vi "Balance Loop.vi"(8 "error in (no error)":errorcluster, 9 "PID gains":T1={"proportional gain (Kc)"=-4.805, "integral time (Ti, min)"=50.38629, "derivative time (Td, min)"=0.000943} {"derivative time (Td, min)" format="%.3f"; "integral time (Ti, min)" format="%.3f"; "proportional gain (Kc)" format="%.3f"}, 10 "maxDiff":dbl=0.75, 11 "Refnum in":refnum<k20>) -> (0 "error out":errorcluster, 3 "Refnum Out":refnum<k20>)   [LabVIEW 2016]
uses:
  <vilib>/Platform/TimedLoop/XDataNode/timing_clust.ctl
  <vilib>/Platform/TimedLoop/XDataNode/nitl_modes.ctl
  <vilib>/Platform/TimedLoop/XDataNode/wakeup.ctl
  Typedef/Remote Control Cluster.ctl
  Typedef/INS Data.ctl
  Shared resoruces/Navigation Variables.vi
  Shared resoruces/Front Panel Control Variables.vi
  <vilib>/addons/control/pid/pid.llb/PID (DBL).vi
  <vilib>/Utility/error.llb/Error Cluster From Error Code.vi
  <vilib>/rvi/errors/niLvFpgaAdjustHostInterfaceError.vi
  <vilib>/RVI Host/nirviSupport.llb/nirviErrorClusterFromErrorCode.vi
  <vilib>/platform/TimedLoop/XDataNode/XDataNode.xnode
  <vilib>/rvi/interface/nirviMethod/nirviMethod.xnode
  <vilib>/rvi/interface/nirviReadWriteControl/nirviReadWriteControl.xnode
  NiFpgaLv.dll
  <vilib>/rvi/interface/Simulation/niFpgaSimulationCallBeginRW.vi
  <vilib>/FPGAPlugInAG/Dynamic/niLvFpga_WriteFifo_Dynamic.vi
  <vilib>/rvi/errors/niLvFpgaMergeErrorWithErrorCode.vi
  <vilib>/rvi/interface/nirviMethod/StockFPGA_InlinedMethodWaitForSingleIRQ.vi
  <vilib>/FPGAPlugInAG/Dynamic/niLvFpga_WaitOnIrq_Dynamic.vi
  <vilib>/FPGAPlugInAG/Dynamic/niLvFpga_AcknowledgeIrq_Dynamic.vi
  <vilib>/addons/control/pid/NI_PID_pid.lvlib
  Shared resoruces/Shared resources RT.lvlib
  <vilib>/Platform/TimedLoop/XDataNode/XDNodeRunTimeDep.lvlib
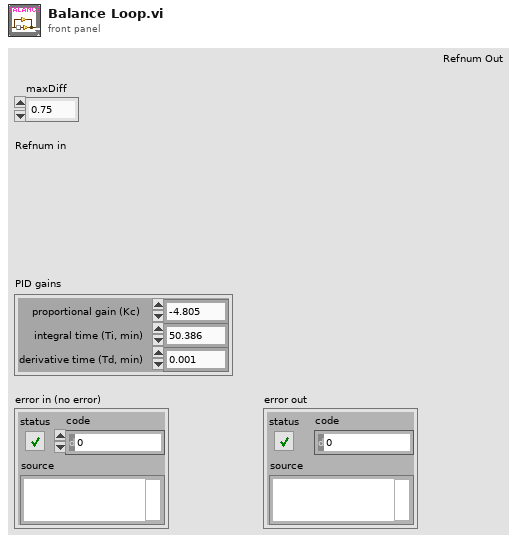
[diagram p1: front panel]
types:
  T1 = cluster{"proportional gain (Kc)":dbl, "integral time (Ti, min)":dbl, "derivative time (Td, min)":dbl}
  T2 = typedef "XDNodeRunTimeDep.lvlib/timing_clust.ctl" = cluster{"Expected End [f-1]":u64, "Actual End [f-1]":u64, "Finished Late? [f-1]":bool, "Expected End [i-1]":u64, "Actual End [i-1]":u64, "Finished Late? [i-1]":bool, "Expected Start [i]":u64, "Actual Start [i]":u64, "Expected Start [f]":u64, "Actual Start [f]":u64, "Source Name":string, "Structure Name":string, "Period":i64, "Deadline":i64, "Offset":i64, "Start":i64, "Priority":i32, "Timeout":i32, "Mode":T3, "Wakeup Reason":T4, "Error":errorcluster, "Source Type":string, "Secondary Source Type":string, "Global End Time":u64, "Global Start Time":u64, "Frame Duration":u64, "Iteration Duration":u64, "Assigned CPU":i32, "I/O Scan Engine Mode":u32}
  T3 = typedef "XDNodeRunTimeDep.lvlib/nitl_modes.ctl" = enum32{"No Change", "Process missed periods, maintain original phase", "Discard missed periods, maintain original phase", "Process missed periods, ignore original phase", "Discard missed periods, ignore original phase"}
  T4 = typedef "XDNodeRunTimeDep.lvlib/wakeup.ctl" = enum32{"Normal", "Aborted", "Asynchronous wakeup", "Timing source error", "Timed loop error", "Timeout"}
  T5 = typedef "Remote Control Cluster.ctl" = cluster{"Pot1":u16, "Pot2":u16, "Pot3":u16, "Pot4":u16, "Switch1":cluster{"L":bool, "H":bool}, "Switch2":cluster{"L":bool, "H":bool}, "Switch3":cluster{"L":bool, "H":bool}}
  T6 = typedef "INS Data.ctl" = cluster{"Yaw":sgl, "Pitch":sgl, "Roll":sgl, "Lat":dbl, "Long":dbl, "Alt":dbl, "North":dbl, "East":dbl, "Down":dbl, "PosU":dbl, "VelU":dbl}
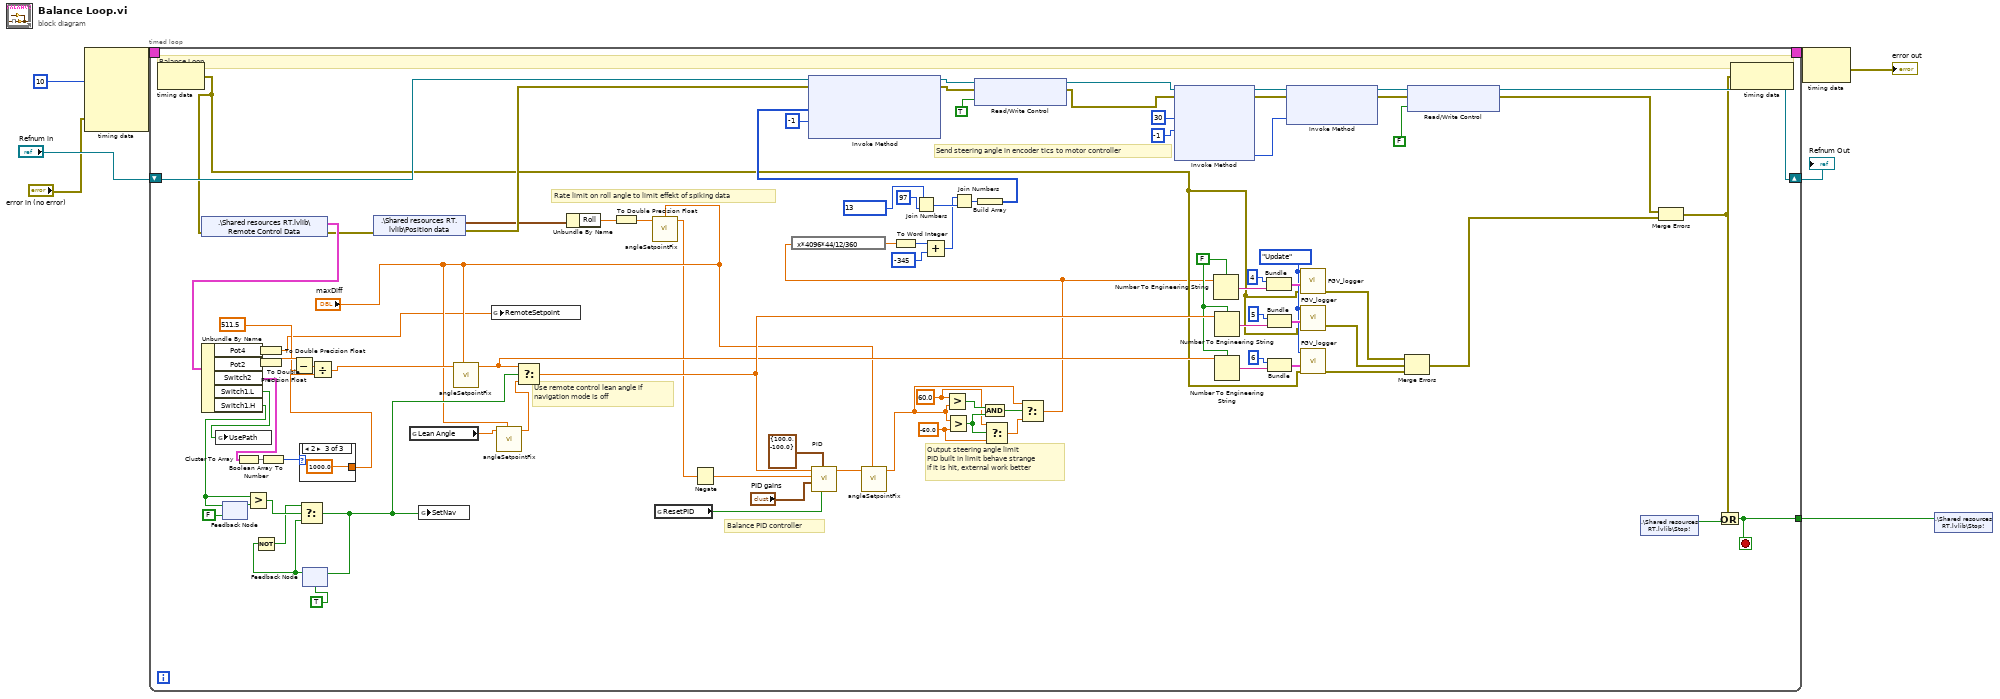
[diagram p0: block diagram]
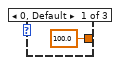
[diagram p2: hidden frame]
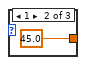
[diagram p3: hidden frame]
diagram:
  n1 = node-c288(i64 10 ("Period"), "error in (no error)") -> (w5:T2)  [unwired: 3 in]
  n2 = timed-loop {
    shift-right: [w97] -> w6
    shift-left: "Refnum in" -> [w98]
    tunnel: [w67] -> w7
    timing: w5 -> [_]
    timing-out: [_] -> w4
    stop <- w67 stop-if-true
    w17 = -60.0
    w18 = 60.0
    w28 = enum16{"Update", "Log", "Init"}."Update" ("Command")
    w32 = FALSE ("use system decimal point (T)")
    # "Use remote control lean angle if \nnavigation mode is off"
    # "Rate limit on roll angle to limit effekt of spiking data"
    # "Output steering angle limit\nPID built in limit behave strange\nif it is hit, external work better"
    # "Balance PID controller"
    # "Send steering angle in encoder tics to motor controller"
    # "Balance Loop"
    n3 = node-c288() -> (w25:errorcluster)  [unwired: 1 in]
    n4 = shared-variable ".\\Shared resources RT.lvlib\\Remote Control Data"(error in=w25) -> (w66:T5, error out=w61:errorcluster)
    n5 = Unbundle By Name(w66) -> ("Pot4"=w23:u16, "Pot2"=w96:u16, "Switch2"=w65:cluster{"L":bool, "H":bool}, "Switch1.L"=w26:bool, "Switch1.H"=w27:bool)
    n6 = global write "Navigation Variables.vi" "UsePath"(w26) -> ()
    n7 = feedback-in #1(w27) -> ()
    n8 = feedback #1(FALSE ("H")) -> (w47:bool)
    n9 = Cluster To Array(cluster=w65) -> (array=w64:bool[])
    n10 = Greater?(x=w27, y=w47) -> (0:w45:bool)
    n11 = To Double Precision Float(number=w23) -> (double precision float=w10:dbl)
    n12 = To Double Precision Float(number=w96) -> (double precision float=w94:dbl)
    n13 = Boolean Array To Number(Boolean array=w64) -> (number=w63:u32)
    n14 = Subtract(x=w94, y=511.5 ("x")) -> (x-y=w95:dbl)
    n15 = case shown="2" w63 {
      tunnel: [100.0 45.0 1000.0] -> w62
      frame 0, Default {
      }
      frame 1 {
      }
      frame 2 {
      }
    }
    n16 = feedback #2(TRUE) -> (w43:bool)
    n17 = Not(x=w43) -> (.not. x?=w42:bool)
    n18 = Select(t=w42, s=w45, f=w43) -> (s? t:f=w36:bool)
    n19 = feedback-in #2(w36) -> ()
    n20 = Divide(x=w95, y=w62) -> (x/y=w30:dbl)
    n21 = shared-variable ".\\Shared resources RT.lvlib\\Position data"(error in=w61) -> (w59:T6, error out=w60:errorcluster)
    n22 = global read "Navigation Variables.vi" "Lean Angle"() -> (w38:dbl)
    n23 = global write "Navigation Variables.vi" "SetNav"(w36) -> ()
    n24 = call "angleSetpointFix.vi"("maxDiff"="maxDiff", "Angle in"=w30) -> ("Angle out"=w29:dbl)  [unwired: 9 in]
    n25 = global write "Navigation Variables.vi" "RemoteSetpoint"(w10) -> ()
    n26 = call "angleSetpointFix.vi"("maxDiff"="maxDiff", "Angle in"=w38) -> ("Angle out"=w37:dbl)  [unwired: 9 in]
    n27 = Select(t=w29, s=w36, f=w37) -> (s? t:f=w40:dbl)
    n28 = Unbundle By Name(w59) -> ("Roll"=w14:sgl)
    n29 = To Double Precision Float(number=w14) -> (double precision float=w11:dbl)
    n30 = call "angleSetpointFix.vi"("maxDiff"="maxDiff", "Angle in"=w11) -> ("Angle out"=w12:dbl)  [unwired: 9 in]
    n31 = global read "Front Panel Control Variables.vi" "ResetPID"() -> (w39:bool)
    n32 = Negate(x=w12) -> (-x=w9:dbl)
    n33 = call-poly <vilib>:"PID.vi"("reinitialize? (F)"=w39, "output range"=cluster{"output high":dbl, "output low":dbl} {"output high"=100.0, "output low"=-100.0}, "PID gains"="PID gains", "process variable"=w9, "setpoint"=w40) -> ("output"=w69:dbl)  [unwired: 5 in, 1 out]
    n34 = call "angleSetpointFix.vi"("maxDiff"="maxDiff", "Angle in"=w69) -> ("Angle out"=w20:dbl)  [unwired: 9 in]
    n35 = Join Numbers(hi=u8 13 ("lo"), lo=u8 97) -> ((hi.lo)=w77:u16)
    n36 = Greater?(x=w18, y=w20) -> (0:w22:bool)
    n37 = Greater?(x=w20, y=w17) -> (0:w19:bool)
    n38 = And(x=w22, y=w19) -> (x .and. y?=w21:bool)
    n39 = Select(t=w18, s=w19, f=w17) -> (s? t:f=w16:dbl)
    n40 = Select(t=w20, s=w21, f=w16) -> (s? t:f=w15:dbl)
    n41 = expression code="x*4096*44/12/360"(w15) -> (w71:dbl)
    n42 = To Word Integer(number=w71) -> (16bit integer=w74:i16)
    n43 = Add(x=w74, y=i16 -345 ("hi")) -> (x+y=w72:i16)
    n44 = Join Numbers(hi=w72, lo=w77) -> ((hi.lo)=w76:u32)
    n45 = Build Array(w76) -> (w73:u32[])
    n46 = xnode "Invoke Method"("FPGA VI Reference In"=w98, "error in"=w60, "Data"=w73, "Timeout (ms)"=-1) -> ("FPGA VI Reference Out"=w85:refnum<k20>, "error out"=w86:errorcluster)  [unwired: 1 out]
    n47 = xnode "Read/Write Control"("FPGA VI Reference In"=w85, "error in"=w86, "ODrive RT Control"=TRUE) -> ("FPGA VI Reference Out"=w84:refnum<k20>, "error out"=w83:errorcluster)
    n48 = xnode "Invoke Method"("FPGA VI Reference In"=w84, "error in"=w83, "IRQ Number(s)"=30, "Timeout (ms)"=-1) -> ("FPGA VI Reference Out"=w92:refnum<k20>, "error out"=w91:errorcluster, "IRQ(s) Asserted"=w81:i32)  [unwired: 1 out]
    n49 = Number To Engineering String(1:w32, 4:w15) -> (0:w56:string)  [unwired: 2 in]
    n50 = Number To Engineering String(1:w32, 4:w40) -> (0:w53:string)  [unwired: 2 in]
    n51 = Number To Engineering String(1:w32, 4:w29) -> (0:w33:string)  [unwired: 2 in]
    n52 = Bundle(4, w56) -> (w57:cluster{i32, string})  [unwired: 1 in]
    n53 = Bundle(5, w53) -> (w54:cluster{i32, string})  [unwired: 1 in]
    n54 = Bundle(6, w33) -> (w34:cluster{i32, string})  [unwired: 1 in]
    n55 = xnode "Invoke Method"("FPGA VI Reference In"=w92, "error in"=w91, "IRQ Number(s)"=w81) -> ("FPGA VI Reference Out"=w89:refnum<k20>, "error out"=w80:errorcluster)
    n56 = call "FGV_logger.vi"("error in"=w25, 9:w57, "Command"=w28) -> ("error out"=w52:errorcluster)  [unwired: 8 in]
    n57 = call "FGV_logger.vi"("error in"=w25, 9:w54, "Command"=w28) -> ("error out"=w51:errorcluster)  [unwired: 8 in]
    n58 = call "FGV_logger.vi"("error in"=w25, 9:w34, "Command"=w28) -> ("error out"=w31:errorcluster)  [unwired: 8 in]
    n59 = Merge Errors(w52, w51, w31) -> (w49:errorcluster)
    n60 = xnode "Read/Write Control"("FPGA VI Reference In"=w89, "error in"=w80, "ODrive RT Control"=FALSE) -> ("FPGA VI Reference Out"=w97:refnum<k20>, "error out"=w50:errorcluster)
    n61 = shared-variable ".\\Shared resources RT.lvlib\\Stop!"() -> (w68:bool)  [unwired: 1 in, 1 out]
    n62 = Merge Errors(w50, w49) -> (w24:errorcluster)
    n63 = Or(x=w24, y=w68) -> (x .or. y?=w67:bool)
    n64 = node-c288(w24) -> ()  [unwired: 1 out]
  }
  "Refnum Out" <- w6
  n65 = node-c288(w4) -> (→"error out":errorcluster)
  n66 = shared-variable ".\\Shared resources RT.lvlib\\Stop!"(w7) -> ()  [unwired: 1 in, 1 out]
